vi "Contour Area.vi"(7 "Oriented? (Default: False)":bool, 8 "error in (no error)":errorcluster, 11 "Points in":T1[](array[typedef])) -> (0 "error out":errorcluster, 3 "Area":dbl)   [LabVIEW 2020, in "shape.lvlib"]
doc: "Compute the Area of a given Contour."
uses:
  shape.lvlib
  common/Image Point (Integer).ctl
  common/common.lvlib
  common/bin/gartoolkit_32-1.dll
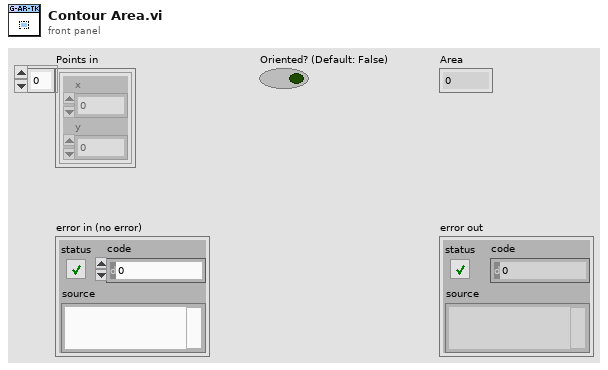
[diagram p1: front panel]
types:
  T1 = typedef "common.lvlib/Image Point (Integer).ctl" = cluster{"x":i32, "y":i32}
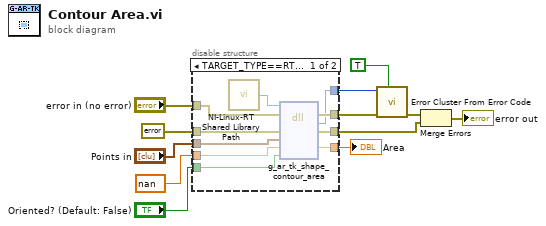
[diagram p0: block diagram]
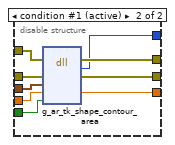
[diagram p2: hidden frame]
diagram:
  n1 = disable-structure shown="TARGET_TYPE==RT&&OS==Linux" {
    disable-tunnel: errorcluster {"status"=FALSE, "code"=0, "source"=""} ("error constant") -> [w18 w31]
    disable-tunnel: "Points in" -> [w19 w30]
    disable-tunnel: nan ("arc_length") -> [w21 w29]
    disable-tunnel: "Oriented? (Default: False)" -> [w22 w28]
    disable-tunnel: [w16 w27] -> w6
    disable-tunnel: [w14 w26] -> w5
    disable-tunnel: [w15 w25] -> w4
    disable-tunnel: [w20 w24] -> w3
    disable-tunnel: "error in (no error)" -> [w17 w23]
    frame condition #0 {
      n2 = call "NI-Linux-RT Shared Library Path.vi"() -> ("Path"=w13:path)
      n3 = dll-call lib="?" fn="g_ar_tk_shape_contour_area" ("g_ar_toolkit.*.*:g_ar_tk_image_draw_line")(path in=w13, error in=w17, "error_cluster"=w18, "points"=w19, "area"=w21, "is_closed"=w22) -> (error out=w16:errorcluster, w14:i32, "error_cluster"=w15:errorcluster, "area"=w20:dbl)  [unwired: 3 in, 1 out]
    }
    frame condition #1 (active) {
      n4 = dll-call lib="C:/serenial/lib/g-augmented-reality-toolkit/LabVIEW/common/bin/gartoolkit_*-1.*" fn="g_ar_tk_shape_contour_area" ("g_ar_toolkit.*.*:g_ar_tk_image_draw_line")(error in=w23, "error_cluster"=w31, "points"=w30, "area"=w29, "is_closed"=w28) -> (error out=w27:errorcluster, w26:i32, "error_cluster"=w25:errorcluster, "area"=w24:dbl)  [unwired: 4 in, 1 out]
    }
  }
  "Area" <- w3
  n5 = call <vilib>:"Error Cluster From Error Code.vi"("show call chain? (False)"=TRUE, "error in (no error)"=w6, "error code (0)"=w5) -> ("error out"=w11:errorcluster)  [unwired: 6 in]
  n6 = Merge Errors(w11, w4) -> (→"error out":errorcluster)
